vi "index_FFT_(freqs,vals).vi"(9 "complex fft":cdb[](array[numeric]), 10 "desired freqs":dbl[](array[numeric]) format="%#_6f", 11 "df":dbl) -> (0 "phase array":dbl[](array[numeric]), 1 "magnitude array":dbl[](array[numeric]), 2 "phase cluster":cluster{"desired freqs":dbl[], dbl[]}, 3 "magnitude cluster":cluster{"desired freqs":dbl[], dbl[]}, 5 "complex array out":cdb[](array[numeric]))   [LabVIEW 2021]
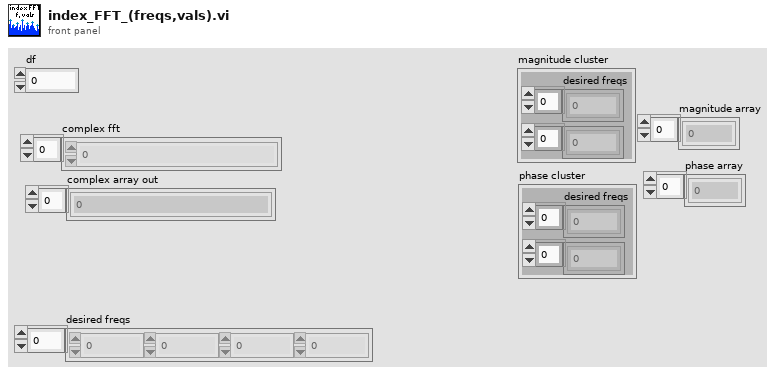
[diagram p1: front panel]
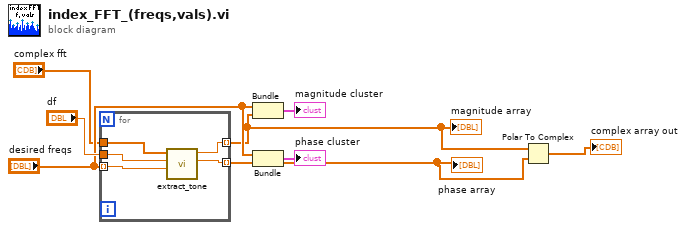
[diagram p0: block diagram]
diagram:
  n1 = for {
    tunnel: "desired freqs" -> [w13] mode=indexing
    tunnel: "df" -> [w12]
    tunnel: "complex fft" -> [w11]
    tunnel: [w10] -> w3 mode=indexing
    tunnel: [w9] -> w2 mode=indexing
    n2 = call "extract_tone.vi"("tone frequency [Hz]"=w13, "df"=w12, "complex fft"=w11) -> ("phase (rad)"=w9:dbl, "amplitude"=w10:dbl)  [unwired: 7 in]
  }
  "phase array" <- w2
  "magnitude array" <- w3
  n3 = Bundle("desired freqs"="desired freqs", w3) -> (→"magnitude cluster":cluster{"desired freqs":dbl[], dbl[]})  [unwired: 1 in]
  n4 = Bundle("desired freqs"="desired freqs", w2) -> (→"phase cluster":cluster{"desired freqs":dbl[], dbl[]})  [unwired: 1 in]
  n5 = Polar To Complex(1:w2, 2:w3) -> (0:→"complex array out":cdb[])
